vi "Set Color Ramp Palette v3.vi"(5 "Image High Color":u32(colorbox), 7 "Image Low Color":u32(colorbox), 8 "error in (no error)":errorcluster, 9 "Image Display Range":cluster{"Min Value":dbl, "Max Value":dbl}={"Min Value"=nan, "Max Value"=nan}, 10 "Image Display Palette Information":T1 {"Palette Type" items=["Grayscale", "Binary", "Gradient", "Rainbow", "Temperature", "User Defined", "Binary 16 Bit", "Gradient 16 Bit", "Rainbow 16 Bit", "Temperature 16 Bit", "User Defined 16 Bit"]}, 11 "ColorRamp in":refnum<vi>) -> (0 "Error Out":errorcluster, 1 "Scale Marker Values":cluster{"Numeric":dbl, "Numeric":u32}[](array[cluster]), 3 "ColorRamp (dup)":refnum<vi>)   [LabVIEW 2021, in "Palette.lvlib"]
uses:
  Palette.lvlib
  Image Palette Information.ctl
  Image/Image Display Palette Type.ctl
  Image/Image.lvlib
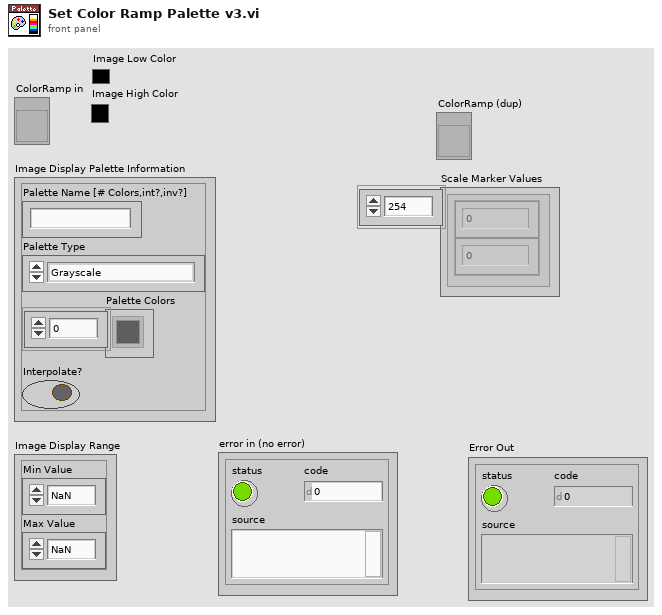
[diagram p1: front panel]
types:
  T1 = typedef "Palette.lvlib/Image Palette Information.ctl" = cluster{"Palette Name [# Colors,int?,inv?]":string, "Palette Type":T2, "Palette Colors":u32[], "Interpolate?":bool}
  T2 = typedef "Image.lvlib/Image Display Palette Type.ctl" = u32
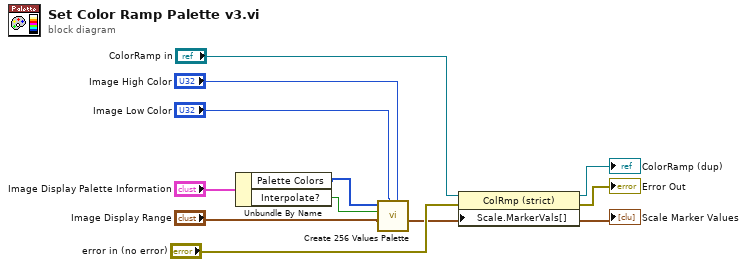
[diagram p0: block diagram]
diagram:
  n1 = Unbundle By Name("Image Display Palette Information") -> ("Palette Colors"=w9:u32[], "Interpolate?"=w8:bool)
  n2 = call "Create 256 Values Palette.vi"("Image High Color"="Image High Color", "Image Low Color"="Image Low Color", "Source Image Display Range"="Image Display Range", "Interpolate?"=w8, "Palette Colors in"=w9) -> ("Color Scale Marker Values"=w1:cluster{"Value":dbl, "Color":u32}[])  [unwired: 3 in, 3 out]
  "Scale Marker Values" <- w1
  n3 = property class="ColRmp (strict)"(reference="ColorRamp in", error in="error in (no error)", "Scale.MarkerVals[]"=w1) -> (reference out=→"ColorRamp (dup)":refnum<vi>, error out=→"Error Out":errorcluster)
